vi "loadHTSummary.vi"() -> ()   [LabVIEW 2012]
uses:
  <vilib>/addons/database/Connection.llb/DB Tools Open Connec (Path).vi
  <vilib>/addons/database/NI_Database_API.lvlib
panel:
  in  "machine":string
  out "error out":errorcluster
  in  "input cluster 2":T1
  out "concatenated string":string
  out "concatenated string 2":string
  out "filenames":string[](array[string])
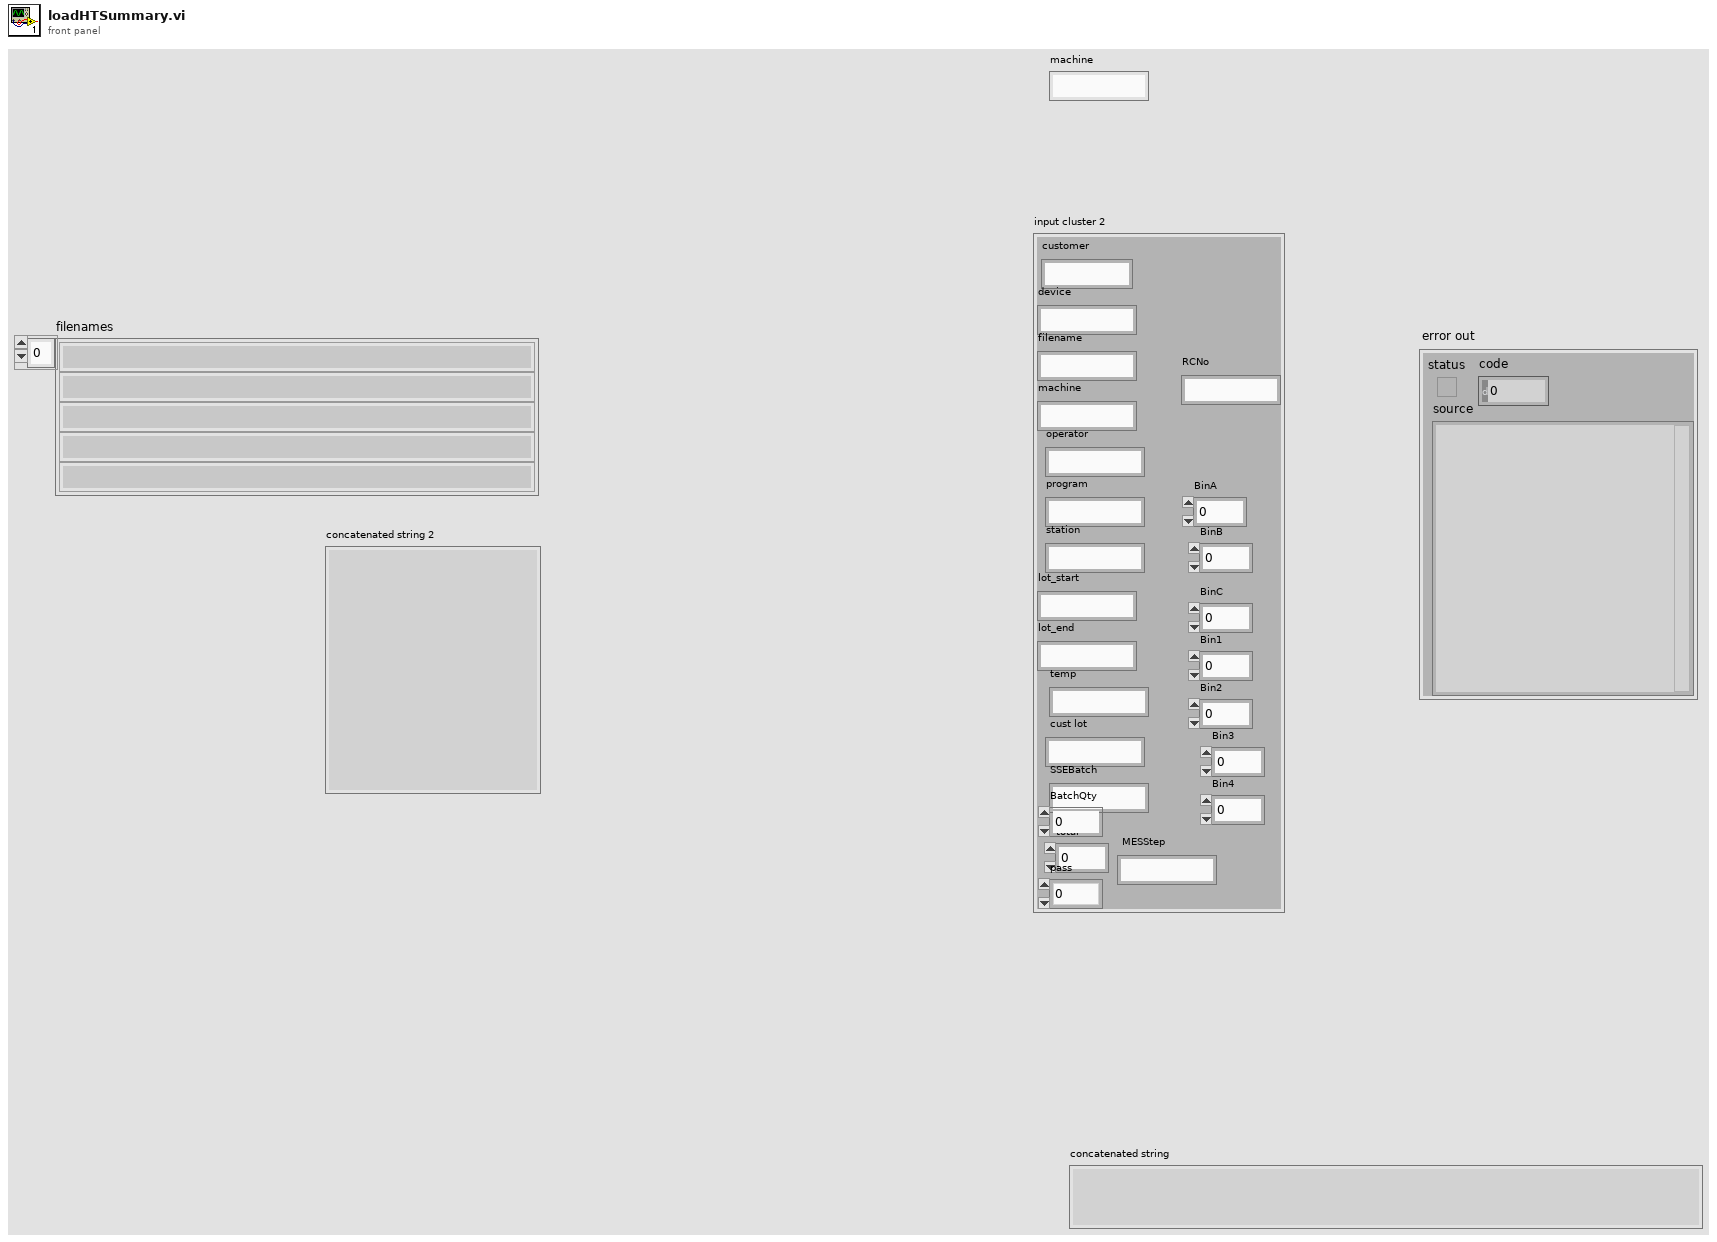
[diagram p1: front panel]
types:
  T1 = cluster{"customer":string, "device":string, "filename":string, "RCNo":string, "machine":string, "operator":string, "program":string, "station":string, "lot_start":string, "lot_end":string, "temp":string, "cust lot":string, "SSEBatch":string, "BatchQty":dbl, "total":dbl, "pass":dbl, "BinA":dbl, "BinB":dbl, "BinC":dbl, "Bin1":dbl, "Bin2":dbl, "Bin3":dbl, "Bin4":dbl, "MESStep":string}
  T2 = typedef "NI_Database_API.lvlib/Conn ObjectReference.ctl" = refnum<k1>
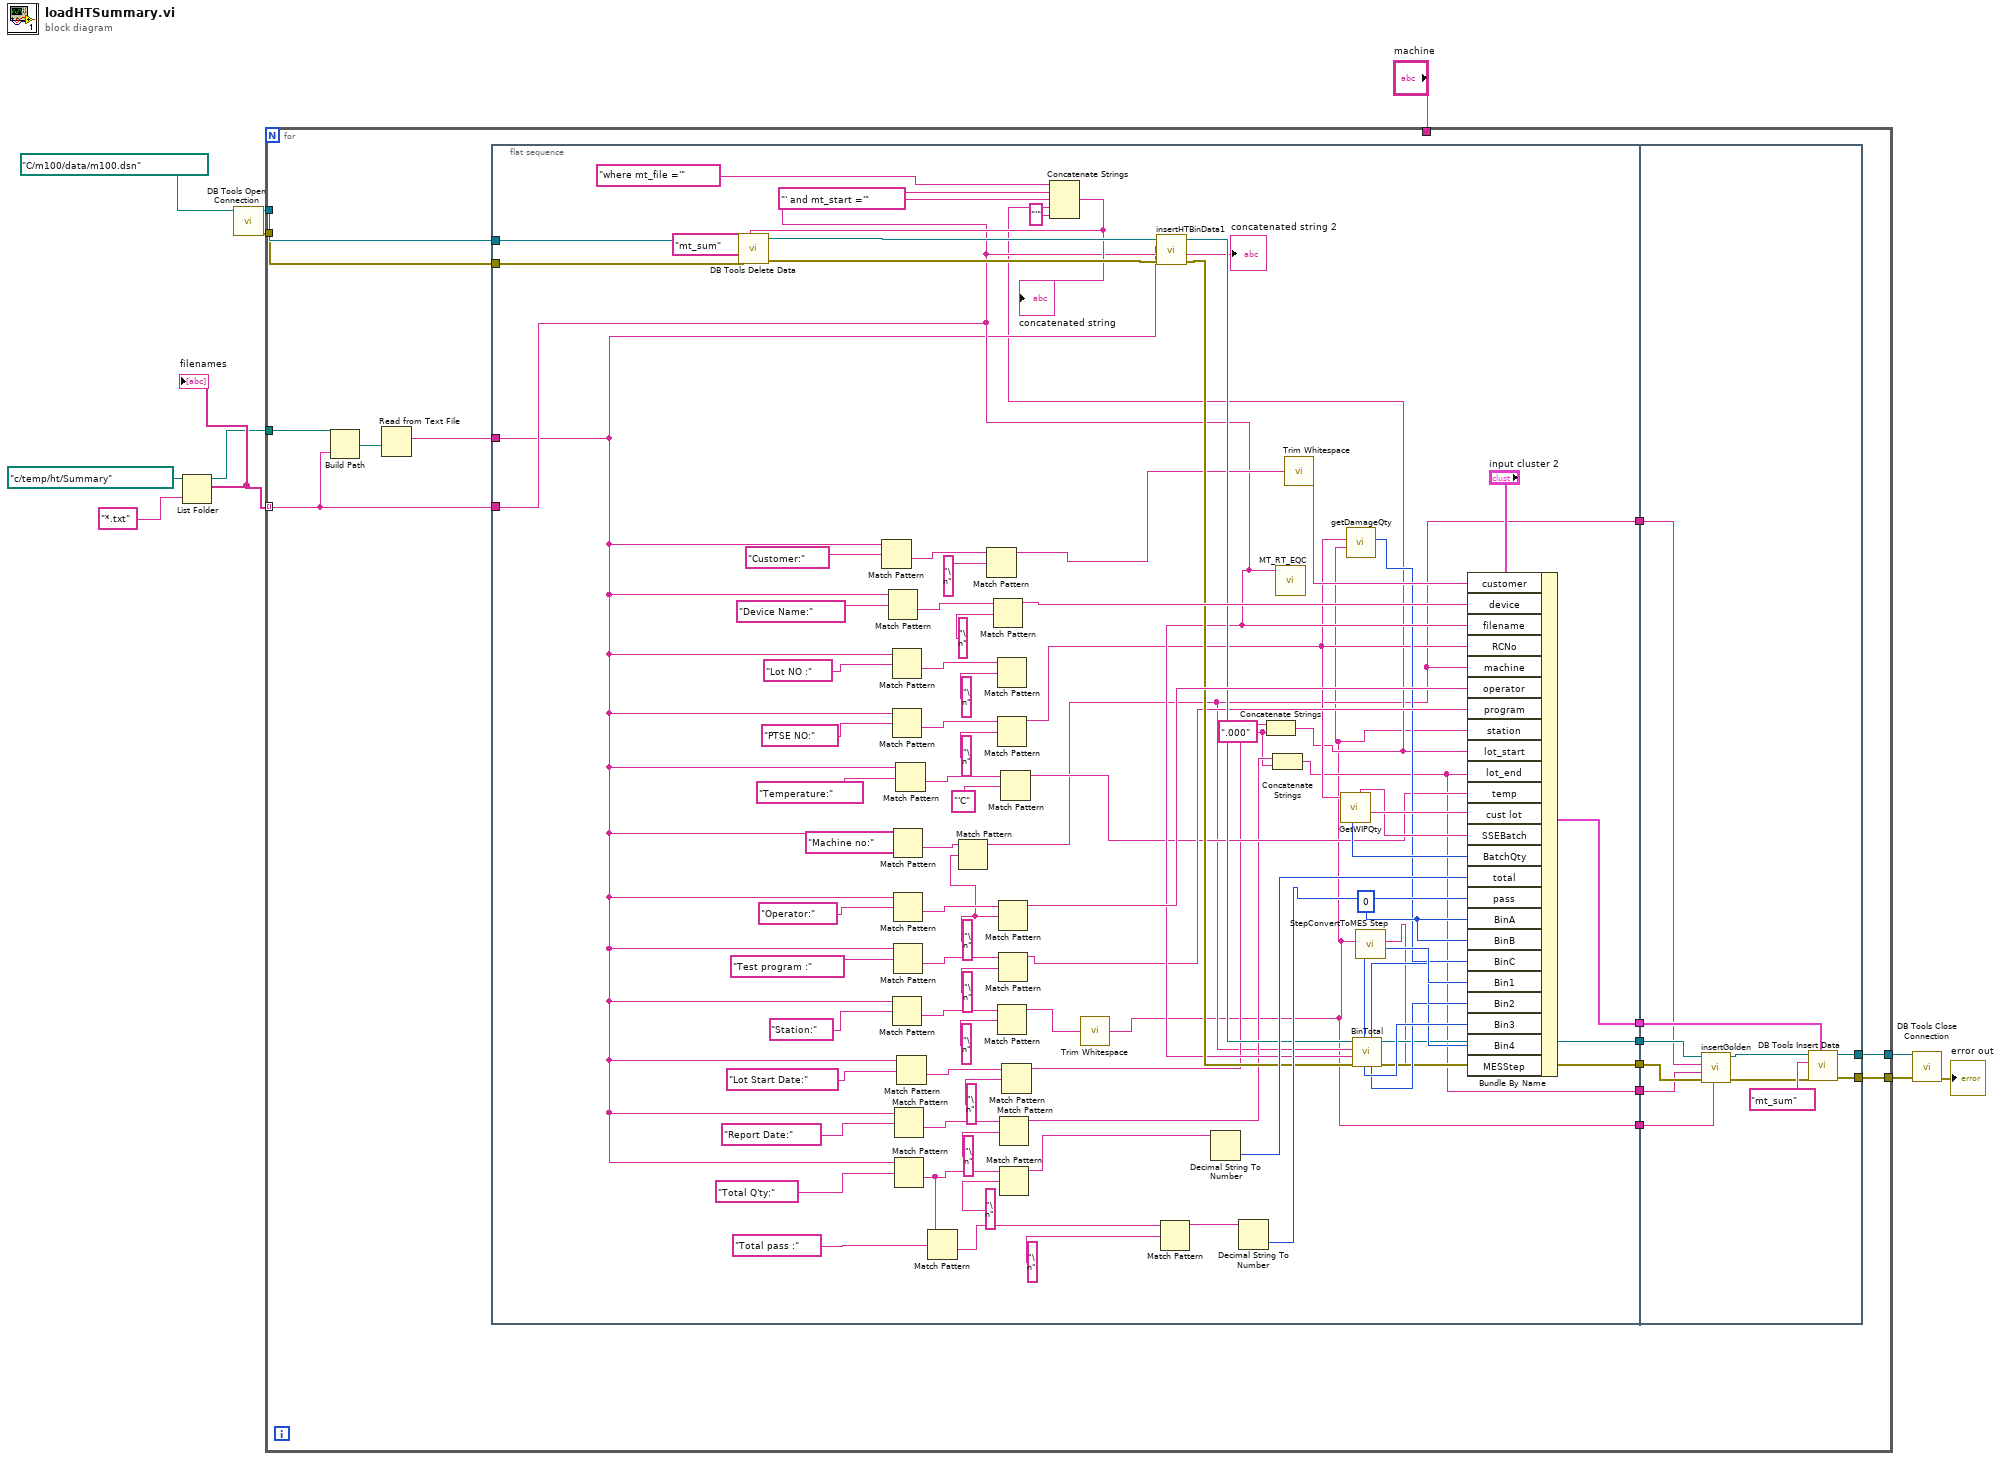
[diagram p0: block diagram]
diagram:
  n1 = List Folder(path=path "c:/temp/ht/Summary", pattern="*.txt") -> (path out=w9:path, filenames=w10:string[])  [unwired: 2 in, 2 out]
  "filenames" <- w10
  n2 = call-poly <vilib>:"DB Tools Open Connection.vi"("connection information"=path "C:/m100/data/m100.dsn") -> ("error out"=w6:errorcluster, "connection reference"=w7:T2)  [unwired: 7 in]
  n3 = for {
    tunnel: w10 -> [w15] mode=indexing
    tunnel: w9 -> [w24]
    tunnel: w7 -> [w23]
    tunnel: w6 -> [w22]
    tunnel: "machine" -> [_]
    tunnel: [w18] -> w3
    tunnel: [w17] -> w2
    n4 = Build Path(base path=w24, name or relative path=w15) -> (appended path=w25:path)
    n5 = Read from Text File(file (use dialog)=w25) -> (text=w21:string)  [unwired: 3 in, 3 out]
    n6 = flat-sequence {
      tunnel: w23 -> [w47]
      tunnel: w22 -> [w46]
      tunnel: w21 -> [w35]
      tunnel: [w54] -> w20
      tunnel: [w53] -> w19
      tunnel: [w42] -> w16
      tunnel: w15 -> [w38]
      tunnel: [w28] -> w14
      tunnel: [w27] -> w13
      tunnel: [w26] -> w12
      tunnel: w20 -> [w115]
      tunnel: w19 -> [w114]
      tunnel: [w120] -> w18
      tunnel: [w119] -> w17
      tunnel: w16 -> [w121]
      tunnel: w14 -> [w113]
      tunnel: w13 -> [w112]
      tunnel: w12 -> [w111]
      frame #0 {
        w29 = ".000" ("string")
        w52 = 0
        w61 = "\n" ("regular expression")
        n7 = Match Pattern(string=w35, regular expression="Customer:") -> (after substring=w109:string)  [unwired: 1 in, 3 out]
        n8 = Match Pattern(string=w35, regular expression="Device Name:") -> (after substring=w106:string)  [unwired: 1 in, 3 out]
        n9 = Match Pattern(string=w35, regular expression="Lot NO :") -> (after substring=w103:string)  [unwired: 1 in, 3 out]
        n10 = Match Pattern(string=w35, regular expression="PTSE NO:") -> (after substring=w100:string)  [unwired: 1 in, 3 out]
        n11 = Match Pattern(string=w35, regular expression="Station:") -> (after substring=w89:string)  [unwired: 1 in, 3 out]
        n12 = Match Pattern(string=w35, regular expression="Machine no:") -> (after substring=w62:string)  [unwired: 1 in, 3 out]
        n13 = Match Pattern(string=w35, regular expression="Operator:") -> (after substring=w94:string)  [unwired: 1 in, 3 out]
        n14 = Match Pattern(string=w35, regular expression="Test program :") -> (after substring=w92:string)  [unwired: 1 in, 3 out]
        n15 = Match Pattern(string=w35, regular expression="Report Date:") -> (after substring=w83:string)  [unwired: 1 in, 3 out]
        n16 = Match Pattern(string=w35, regular expression="Total Q'ty:") -> (after substring=w79:string)  [unwired: 1 in, 3 out]
        n17 = Match Pattern(string=w35, regular expression="Temperature:") -> (after substring=w97:string)  [unwired: 1 in, 3 out]
        n18 = Match Pattern(string=w35, regular expression="Lot Start Date:") -> (after substring=w86:string)  [unwired: 1 in, 3 out]
        n19 = Match Pattern(string=w79, regular expression="Total pass :") -> (after substring=w76:string)  [unwired: 1 in, 3 out]
        n20 = Match Pattern(string=w62, regular expression=w61) -> (before substring=w28:string)  [unwired: 1 in, 3 out]
        n21 = Match Pattern(string=w109, regular expression="\n") -> (before substring=w41:string)  [unwired: 1 in, 3 out]
        n22 = Match Pattern(string=w106, regular expression="\n") -> (before substring=w73:string)  [unwired: 1 in, 3 out]
        n23 = Match Pattern(string=w103, regular expression="\n") -> ()  [unwired: 1 in, 4 out]
        n24 = Match Pattern(string=w100, regular expression="\n") -> (before substring=w34:string)  [unwired: 1 in, 3 out]
        n25 = Match Pattern(string=w89, regular expression="\n") -> (before substring=w39:string)  [unwired: 1 in, 3 out]
        n26 = Match Pattern(string=w94, regular expression=w61) -> (before substring=w72:string)  [unwired: 1 in, 3 out]
        n27 = Match Pattern(string=w92, regular expression="\n") -> (before substring=w37:string)  [unwired: 1 in, 3 out]
        n28 = Match Pattern(string=w83, regular expression="\n") -> (before substring=w30:string)  [unwired: 1 in, 3 out]
        n29 = Match Pattern(string=w79, regular expression="\n") -> (before substring=w75:string)  [unwired: 1 in, 3 out]
        n30 = Match Pattern(string=w97, regular expression="'C") -> (before substring=w33:string)  [unwired: 1 in, 3 out]
        n31 = Match Pattern(string=w86, regular expression="\n") -> (before substring=w32:string)  [unwired: 1 in, 3 out]
        n32 = call <vilib>:"Trim Whitespace.vi"("string"=w39) -> ("trimmed string"=w26:string)  [unwired: 1 in]
        n33 = Match Pattern(string=w76, regular expression="\n") -> (before substring=w71:string)  [unwired: 1 in, 3 out]
        n34 = Decimal String To Number(string=w75) -> (number=w68:i32)  [unwired: 2 in, 1 out]
        n35 = Decimal String To Number(string=w71) -> (number=w69:i32)  [unwired: 2 in, 1 out]
        n36 = Concatenate Strings(w32, w29) -> (w31:string)
        n37 = Concatenate Strings("where mt_file ='" ("SQL query"), w38, "' and mt_start ='" ("string"), w31, "'" ("string")) -> (w44:string)
        "concatenated string" <- w44
        n38 = call <vilib>:"DB Tools Delete Data.vi"("condition"=w44, "error in (no error)"=w46, "table"="mt_sum", "connection reference"=w47) -> ("error out"=w48:errorcluster, "connection reference out"=w49:T2)  [unwired: 6 in]
        n39 = call "insertHTBinData1.vi"("error in (no error)"=w48, "FileName"=w38, "String"=w35, "connection reference"=w49) -> ("error out"=w56:errorcluster, "concatenated string"=→"concatenated string 2":string, "connection reference out"=w55:T2)  [unwired: 5 in]
        n40 = Concatenate Strings(w30, w29) -> (w27:string)
        n41 = call "MT_RT_EQC.vi"("input string"=w38) -> ()  [unwired: 6 in, 5 out]
        n42 = call <vilib>:"Trim Whitespace.vi"("string"=w41) -> ("trimmed string"=w40:string)  [unwired: 1 in]
        n43 = call "GetWIPQty.vi"("Lotno"=w34) -> ("lotno"=w70:string, "SSEBATCH"=w66:string, "BATCHQTY"=w67:i32)  [unwired: 2 in, 6 out]
        n44 = call "getDamageQty.vi"("Step"=w26, "RCNo"=w34) -> ("Damage"=w36:i32)  [unwired: 9 in]
        n45 = call "BinTotal.vi"("error out 2"=w56, "fileName"=w38, "machine"=w28, "connection reference"=w55) -> ("error out"=w53:errorcluster, "connection reference 2"=w54:T2, "bin4"=w57:i32, "bin2"=w59:i32, "bin3"=w58:i32, "bin1"=w60:i32)  [unwired: 2 in]
        n46 = call "StepConvertToMES Step.vi"("Step"=w26) -> ("MES Step"=w43:string)  [unwired: 10 in]
        n47 = Bundle By Name(cluster="input cluster 2", "customer"=w40, "device"=w73, "filename"=w38, "RCNo"=w34, "machine"=w28, "operator"=w72, "program"=w37, "station"=w26, "lot_start"=w31, "lot_end"=w27, "temp"=w33, "cust lot"=w70, "SSEBatch"=w66, "BatchQty"=w67, "total"=w68, "pass"=w69, "BinA"=w52, "BinB"=w52, "BinC"=w36, "Bin1"=w60, "Bin2"=w59, "Bin3"=w58, "Bin4"=w57, "MESStep"=w43) -> (w42:T1)
      }
      frame #1 {
        n48 = call "insertGolden.vi"("Station"=w111, "error in (no error)"=w114, "trans_time"=w112, "machine"=w113, "connection reference"=w115) -> ("error out"=w117:errorcluster, "connection reference 2"=w116:T2)  [unwired: 5 in]
        n49 = call <vilib>:"DB Tools Insert Data.vi"("data"=w121, "error in (no error)"=w117, "table"="mt_sum", "connection reference"=w116) -> ("error out"=w119:errorcluster, "connection reference out"=w120:T2)  [unwired: 6 in]
      }
    }
  }
  n50 = call <vilib>:"DB Tools Close Connection.vi"("error in (no error)"=w2, "connection reference"=w3) -> ("error out"=→"error out":errorcluster)  [unwired: 5 in]
